vi "Tracepoint_ManageDrive.vi"(7 "Qbus in":refnum<class "Qbus.lvclass">, 8 "error in (no error)":errorcluster, 9 "free disk space":dbl, 10 "streams deleted":i32, 11 "files deleted":i32) -> (0 "error out":errorcluster)   [LabVIEW 2017, in "FileManager.lvlib"]
uses:
  <vilib>/addons/InsightCM/Devices/Shared/Common/FileManager/FileManager.lvlib
  <vilib>/addons/Qbus/Qbus.lvclass
  <vilib>/addons/TraceLogger/TraceLogger.lvlib
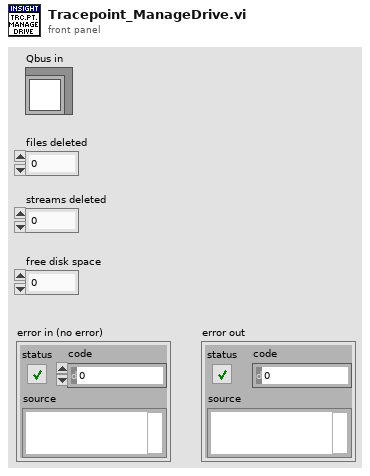
[diagram p1: front panel]
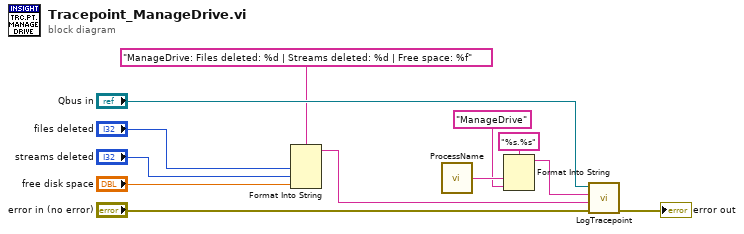
[diagram p0: block diagram]
diagram:
  n1 = Format Into String(format string="ManageDrive: Files deleted: %d | Streams deleted: %d | Free space: %f", "files deleted", "streams deleted", "free disk space") -> (resulting string=w2:string)  [unwired: 2 in, 1 out]
  n2 = call <vilib>:"ProcessName.vi"() -> ("process name"=w9:string)  [unwired: 5 in]
  n3 = Format Into String(format string="%s.%s", w9, "ManageDrive" ("tracepoint")) -> (resulting string=w3:string)  [unwired: 2 in, 1 out]
  n4 = call <vilib>:"LogTracepoint.vi"("error in (no error)"="error in (no error)", "log string"=w2, "tracepoint"=w3, "qbus in"="Qbus in") -> ("error out"=→"error out":errorcluster)  [unwired: 6 in, 1 out]
